vi "APT homing.vi"(8 "error in (no error)":errorcluster, 10 "Boolean in":bool, 11 "Automation Refnum in":refnum<k7>) -> (0 "error out":errorcluster, 2 "Boolean out":bool, 3 "Automation Refnum out":refnum<k7>)   [LabVIEW 2023]
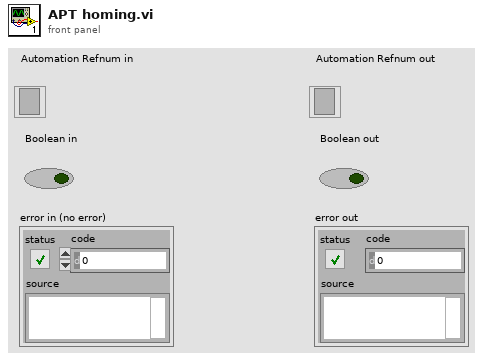
[diagram p1: front panel]
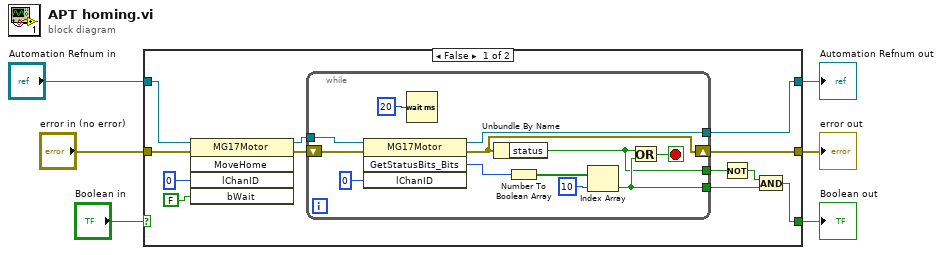
[diagram p0: block diagram]
diagram:
  n1 = case shown="False" "Boolean in" {
    selector: "Boolean in" -> [_ w32]
    tunnel: "Automation Refnum in" -> [w12 w31]
    tunnel: "error in (no error)" -> [w11 w33]
    tunnel: [w8 w33] -> w5
    tunnel: [w10 w32] -> w6
    tunnel: [w9 w31] -> w4
    frame False {
      n2 = invoke class="MG17Motor" method="MoveHome"(reference=w12, error in=w11, "lChanID"=0, "bWait"=FALSE) -> (reference out=w17:refnum<k7>, error out=w16:errorcluster)  [unwired: 1 in, 3 out]
      n3 = while {
        tunnel: w17 -> [w30]
        shift-right: [w24] -> w8
        shift-left: w16 -> [w29]
        tunnel: [w21] -> w9
        tunnel: [w20] -> w15
        tunnel: [w19] -> w13
        stop <- w23 stop-if-true
        n4 = invoke class="MG17Motor" method="GetStatusBits_Bits"(reference=w30, error in=w29, "lChanID"=0) -> (reference out=w21:refnum<k7>, error out=w24:errorcluster, "GetStatusBits_Bits"=w27:i32)  [unwired: 1 in, 1 out]
        n5 = Wait (ms)(milliseconds to wait=u32 20) -> ()  [unwired: 1 out]
        n6 = Unbundle By Name(w24) -> ("status"=w19:bool)
        n7 = Number To Boolean Array(number=w27) -> (Boolean array=w26:bool[])
        n8 = Index Array(array=w26, index=10) -> (element=w20:bool)
        n9 = Or(x=w19, y=w20) -> (x .or. y?=w23:bool)
      }
      n10 = Not(x=w13) -> (.not. x?=w14:bool)
      n11 = And(x=w14, y=w15) -> (x .and. y?=w10:bool)
    }
    frame True {
    }
  }
  "Boolean out" <- w6
  "error out" <- w5
  "Automation Refnum out" <- w4
